vi "ProgramSequence.vi"(10 "Angle":dbl=0.25 min=0.0 step=0.1 format="%#_6p", 11 "Cluster":T1={"Radius"=0.0, "No. of Points"=0, "Center"={"X"=0.0, "Y"=0.0}, "Circle"=FALSE, "Density"=0.0, "PointSpec"=enum."No. Of Points", "Hold"=FALSE, "Size"=1, "LatC"=10.0, "Eccentricity"=0.0, "Phase"=0.0} {"Eccentricity" min=0.0; "Size" step=1; "LatC" step=0.05}) -> (3 "Sequence":dbl[][][](array[numeric]))   [LabVIEW 2017]
uses:
  CircleControls.ctl
panel:
  out "Array 2":dbl[][][](array[numeric])
  out "Array":dbl[][][](array[numeric])
  in  "Delta":dbl=0.2 min=0.0 step=0.1 format="%#_6p"
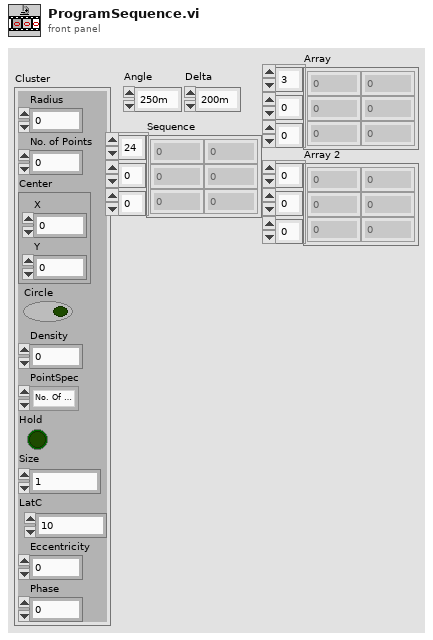
[diagram p1: front panel]
types:
  T1 = typedef "CircleControls.ctl" = cluster{"Radius":dbl, "No. of Points":i32, "Center":cluster{"X":dbl, "Y":dbl}, "Circle":bool, "Density":dbl, "PointSpec":enum32{"No. Of Points", "Density"}, "Hold":bool, "Size":i32, "LatC":dbl, "Eccentricity":dbl, "Phase":dbl}
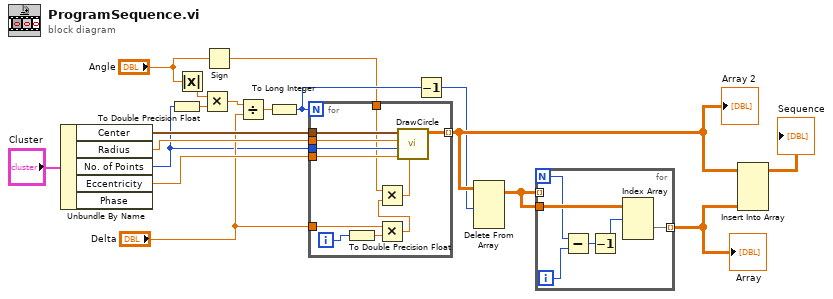
[diagram p0: block diagram]
diagram:
  n1 = Unbundle By Name("Cluster") -> ("Center"=w17:cluster{"X":dbl, "Y":dbl}, "Radius"=w16:dbl, "No. of Points"=w11:i32, "Eccentricity"=w15:dbl)  [unwired: 1 out]
  n2 = To Double Precision Float(number=w11) -> (double precision float=w12:dbl)
  n3 = Absolute Value(x="Angle") -> (abs(x)=w1:dbl)
  n4 = Multiply(x=w1, y=w12) -> (x*y=w14:dbl)
  n5 = Sign(1:"Angle") -> (0:w3:dbl)
  n6 = Divide(x=w14, y="Delta") -> (x/y=w10:dbl)
  n7 = To Long Integer(number=w10) -> (32bit integer=w5:i32)
  n8 = for {
    N: w5 -> [_]
    tunnel: w17 -> [w29]
    tunnel: w16 -> [w28]
    tunnel: w11 -> [w27]
    tunnel: w15 -> [w26]
    tunnel: "Delta" -> [w25]
    tunnel: [w24] -> w8 mode=indexing
    tunnel: w3 -> [w21]
    i -> [w23]
    n9 = To Double Precision Float(number=w23) -> (double precision float=w22:dbl)
    n10 = Multiply(x=w25, y=w22) -> (x*y=w20:dbl)
    n11 = Multiply(x=w21, y=w20) -> (x*y=w19:dbl)
    n12 = call "DrawCircle.vi"("Phase"=w19, "Eccentricity"=w26, "No Of Points"=w27, "Radius"=w28, "Center"=w29) -> ("Array"=w24:dbl[][])  [unwired: 6 in]
  }
  "Array 2" <- w8
  n13 = Decrement(x=w5) -> (x-1=w4:i32)
  n14 = Delete From Array(array=w8, index (dim 0)=w4) -> (array with subset deleted=w9:dbl[][][])  [unwired: 3 in, 1 out]
  n15 = for {
    N -> [w32]
    tunnel: w9 -> [_] mode=indexing
    tunnel: w9 -> [w35]
    tunnel: [w34] -> w7 mode=indexing
    i -> [w33]
    n16 = Subtract(x=w32, y=w33) -> (x-y=w31:i32)
    n17 = Decrement(x=w31) -> (x-1=w30:i32)
    n18 = Index Array(array=w35, index (dim 0)=w30) -> (element=w34:dbl[][])  [unwired: 2 in]
  }
  "Array" <- w7
  n19 = Insert Into Array(array=w8, new element=w7) -> (→"Sequence":dbl[][][])  [unwired: 3 in]
